vi "Set Interval.vi"(8 "error in (no error)":errorcluster, 10 "Interval (ms)":dbl, 11 "Synchronization Device in":refnum<class "NI DAQ.lvclass">) -> (0 "error out":errorcluster, 3 "Synchronization Device out":refnum<class "NI DAQ.lvclass">)   [LabVIEW 2023, in "NI DAQ.lvlib" / "NI DAQ.lvclass"]
uses:
  NI DAQ.lvclass
  NI DAQ.lvclass/NI DAQ.ctl
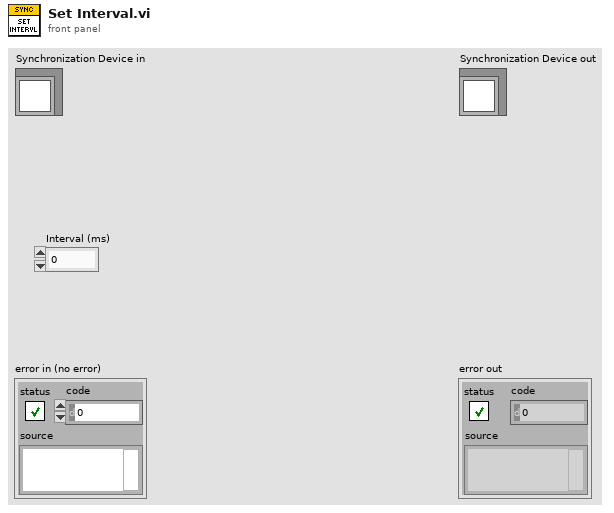
[diagram p1: front panel]
types:
  T1 = typedef "sync device settings.ctl" = cluster{"Interval (ms)":dbl, "ALEX":bool, "Shutter Enable":bool[], "Stream":bool, "Duty Cycle":dbl, "fluidics trigger frame":u16, "Frames to Skip":u32}
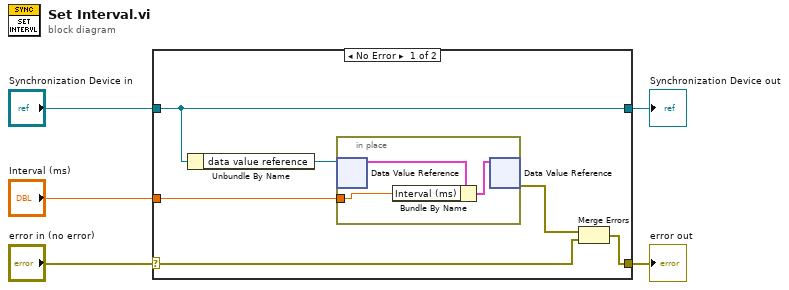
[diagram p0: block diagram]
diagram:
  n1 = case shown="No Error" "error in (no error)" {
    selector: "error in (no error)" -> [w9 w16]
    tunnel: [w10 w16] -> w4
    tunnel: [w11 w15] -> w2
    tunnel: "Synchronization Device in" -> [w11 w15]
    tunnel: "Interval (ms)" -> [w7 _]
    frame No Error {
      n2 = Unbundle By Name(w11) -> ("data value reference"=w8:refnum<data-value>)
      n3 = in-place {
        in-place-border: w7 -> [w12]
        n4 = in-place-dvr #1(w8) -> (w13:T1)  [unwired: 1 out]
        n5 = Bundle By Name(cluster=w13, "Interval (ms)"=w12) -> (w14:T1)
        n6 = in-place-dvr #1(w14) -> (w6:errorcluster)  [unwired: 1 out]
      }
      n7 = Merge Errors(w6, w9) -> (w10:errorcluster)
    }
    frame Error {
    }
  }
  "error out" <- w4
  "Synchronization Device out" <- w2
